vi "Build Folder Report.vi"(0 "directory info in":T1={"target dir"=path "C:/ADIBitbucket/nists19.0_templateproject/Code Modules/Common/Instrument Control/DCPower", "output dir"={"base dir"=path "../docs", "image dir"=path "../docs", "html dir"=path "../docs", "md dir"=path "../docs"}, "folder names"=[], "filenames"=[]}, 7 "Initial Call":bool, 11 "error in":errorcluster) -> (4 "directory info out":T1={"target dir"=path "C:/ADIBitbucket/nists19.0_templateproject/Code Modules/Common/Instrument Control/DCPower", "output dir"={"base dir"=path "../docs", "image dir"=path "../docs", "html dir"=path "../docs", "md dir"=path "../docs"}, "folder names"=[], "filenames"=[]}, 15 "error out":errorcluster)   [LabVIEW 2019, in "MD Generator.lvlib"]
uses:
  MD Generator.lvlib
  Report Path Cluster.ctl
panel:
  out "output file path":path
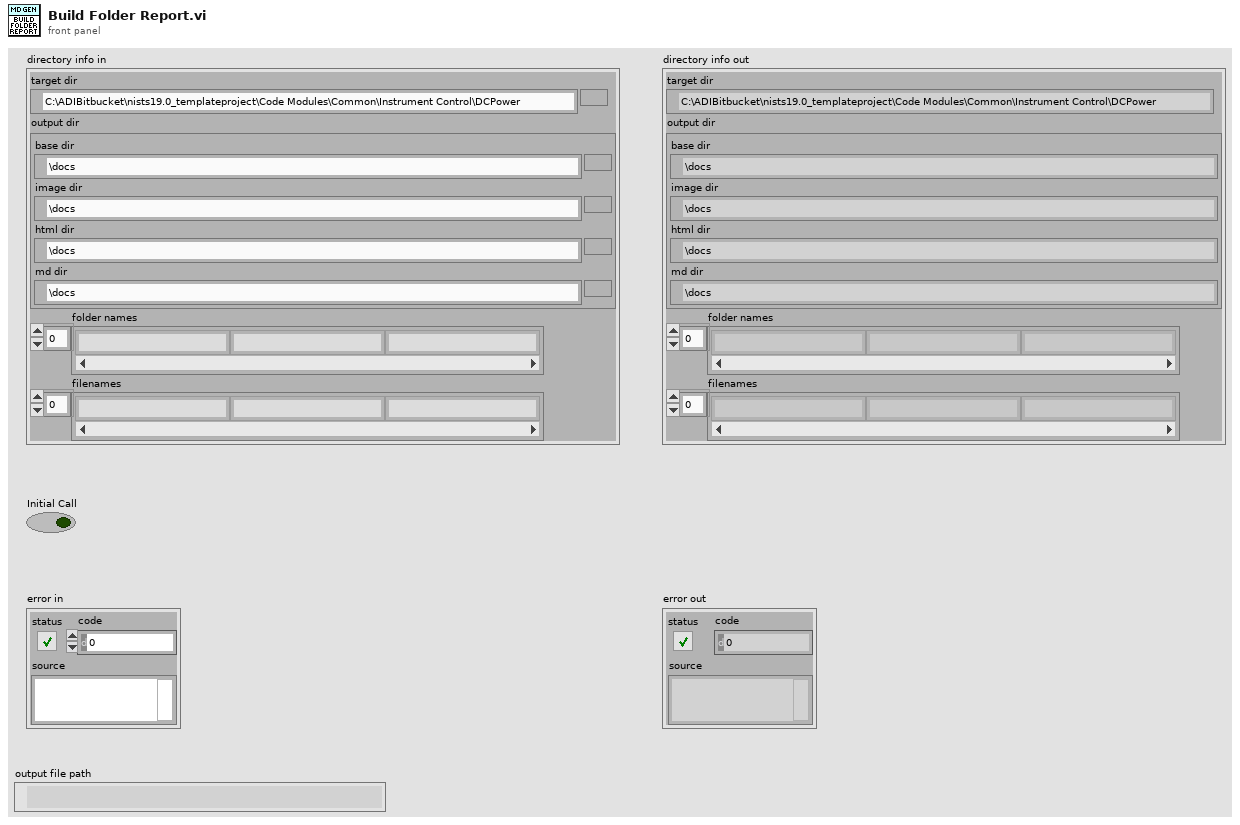
[diagram p1: front panel]
types:
  T1 = typedef "Report Path Cluster.ctl" = cluster{"target dir":path, "output dir":cluster{"base dir":path, "image dir":path, "html dir":path, "md dir":path}, "folder names":string[], "filenames":string[]}
  T2 = enum16{"open", "replace", "create", "open or create", "replace or create", "replace or create with confirmation"}
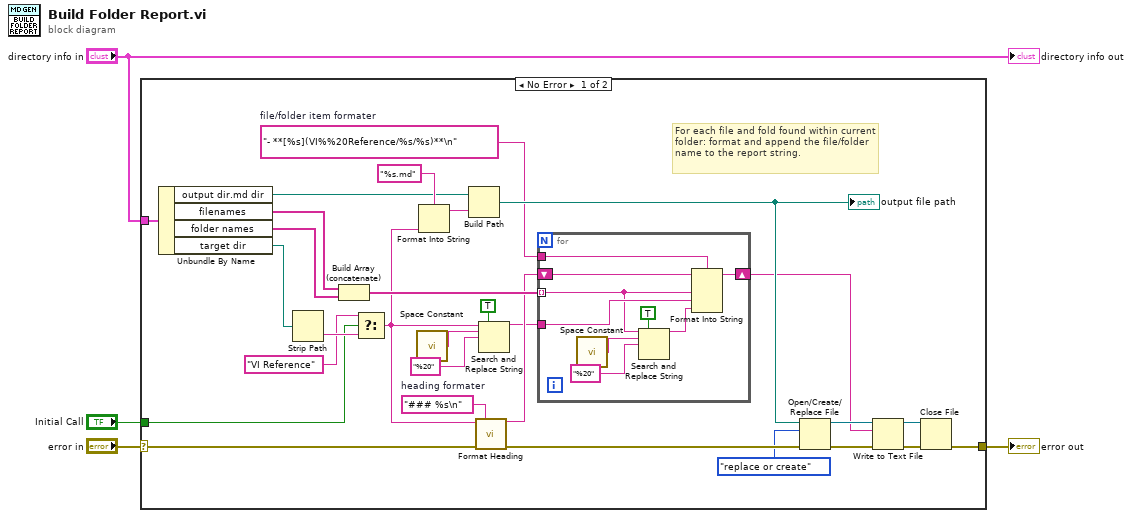
[diagram p0: block diagram]
diagram:
  n1 = case shown="No Error" "error in" {
    selector: "error in" -> [w28 w43]
    tunnel: [w24 w43] -> w3
    tunnel: "directory info in" -> [w31 _]
    tunnel: "Initial Call" -> [w11 _]
    frame No Error {
      w16 = "- **[%s](VI%%20Reference/%s/%s)**\n"  # file/folder item formater
      w17 = "### %s\n"  # heading formater
      # "For each file and fold found within current folder: format and append the file/folder name to the report string."
      n2 = Unbundle By Name(w31) -> ("output dir.md dir"=w29:path, "filenames"=w27:string[], "folder names"=w19:string[], "target dir"=w12:path)
      n3 = Strip Path(path=w12) -> (name=w33:string)  [unwired: 1 out]
      n4 = Build Array (concatenate)(w27, w19) -> (w20:string[])
      n5 = Select(t="VI Reference", s=w11, f=w33) -> (s? t:f=w6:string)
      n6 = call <vilib>:"Space Constant.vi"() -> ("String"=w9:string)
      n7 = Format Into String(format string="%s.md", w6) -> (resulting string=w30:string)  [unwired: 2 in, 1 out]
      n8 = Build Path(base path=w29, name or relative path=w30) -> (appended path=w21:path)
      "output file path" <- w21
      n9 = call "Format Heading.vi"("new heading"=w6, "format string"=w17, "error in"=w28) -> ("string out"=w13:string, "error out"=w15:errorcluster)  [unwired: 11 in]
      n10 = Search and Replace String(replace all?=TRUE ("replace all? (F)"), input string=w6, search string=w9, replace string="%20" ("replace string (\"\")")) -> (result string=w5:string)  [unwired: 4 in, 3 out]
      n11 = for {
        tunnel: w20 -> [w34] mode=indexing
        shift-right: [w41] -> w18
        shift-left: w13 -> [w42]
        tunnel: w16 -> [w40]
        tunnel: w5 -> [w39]
        n12 = call <vilib>:"Space Constant.vi"() -> ("String"=w36:string)
        n13 = Search and Replace String(replace all?=TRUE ("replace all? (F)"), input string=w34, search string=w36, replace string="%20" ("replace string (\"\")")) -> (result string=w35:string)  [unwired: 4 in, 3 out]
        n14 = Format Into String(format string=w40, initial string=w42, w34, w39, w35) -> (resulting string=w41:string)  [unwired: 1 in, 1 out]
      }
      n15 = Open/Create/Replace File(file path (use dialog)=w21, error in=w15, operation (0:open)=T2."replace or create") -> (refnum out=w23:refnum<file>, error out=w26:errorcluster)  [unwired: 3 in, 1 out]
      n16 = Write to Text File(file (use dialog)=w23, text=w18, error in=w26) -> (refnum out=w22:refnum<file>, error out=w25:errorcluster)  [unwired: 1 in, 1 out]
      n17 = Close File(refnum=w22, error in=w25) -> (error out=w24:errorcluster)  [unwired: 1 out]
    }
    frame Error {
    }
  }
  "error out" <- w3
  "directory info out" <- "directory info in"
